vi "探头窗口-12.vi"() -> ()   [LabVIEW 2017]
panel:
  in  "更新数据":T1
  in  "停止信号":bool=TRUE
  out "更新数据？":bool=TRUE
  out "引用-切回列表模式？":refnum<vi>
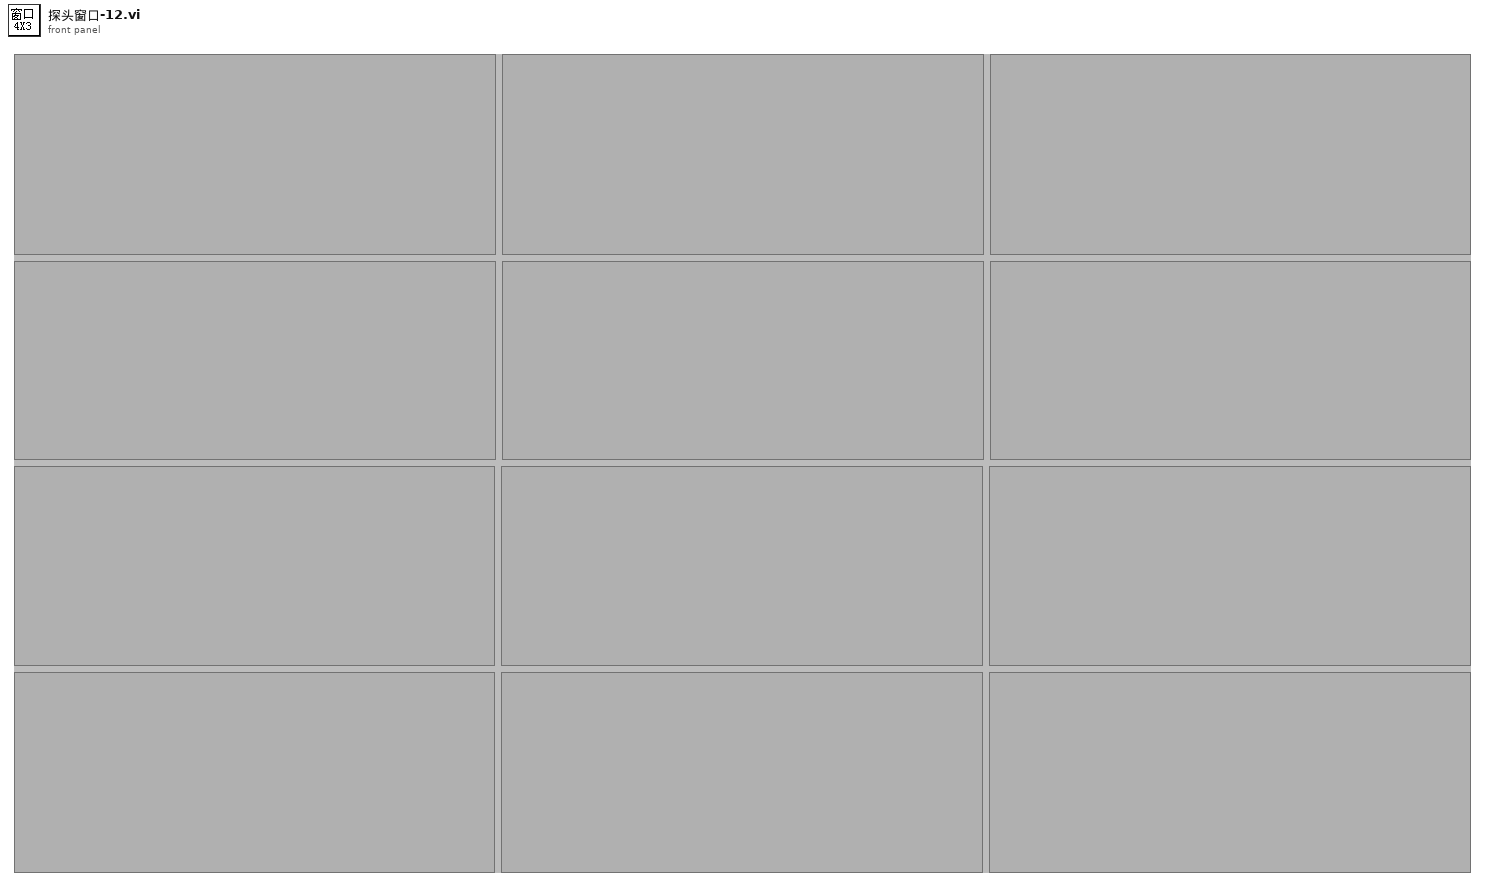
[diagram p1: front panel]
types:
  T1 = cluster{"探头启用状态？":bool[], "测量值":cluster{"X":timestamp, "Y":dbl}[], "限值":cluster{"限值1":dbl, "限值2":dbl, "探头限值":enum16{"一级限值", "二级限值"}}[], "报警状态":enum16{"正常", "一级报警", "二级报警", "累积报警"}[], "探头信息":string[], "累积剂量":cluster{"设备名称":string, "启用累积？":bool, "起始时间":timestamp, "累积剂量":dbl, "累积报警阈值":dbl}[]}
  T2 = cluster{"启用状态？":bool, "测量值":cluster{"X":timestamp, "Y":dbl}, "限值簇":cluster{"限值1":dbl, "限值2":dbl, "探头限值":enum16{"一级限值", "二级限值"}}, "报警状态":enum16{"正常", "一级报警", "二级报警", "累积报警"}, "探头信息":string, "探头地址":i32, "累积剂量":cluster{"设备名称":string, "启用累积？":bool, "起始时间":timestamp, "累积剂量":dbl, "累积报警阈值":dbl}}
  T3 = cluster{"限值1":dbl, "限值2":dbl, "探头限值":enum16{"一级限值", "二级限值"}}
  T4 = cluster{"限值1":dbl, "限值2":dbl, "探头限值":enum16{"一级限值", "二级限值"}}[]
  T5 = cluster{"设备名称":string, "启用累积？":bool, "起始时间":timestamp, "累积剂量":dbl, "累积报警阈值":dbl}[]
  T6 = cluster{"设备名称":string, "启用累积？":bool, "起始时间":timestamp, "累积剂量":dbl, "累积报警阈值":dbl}
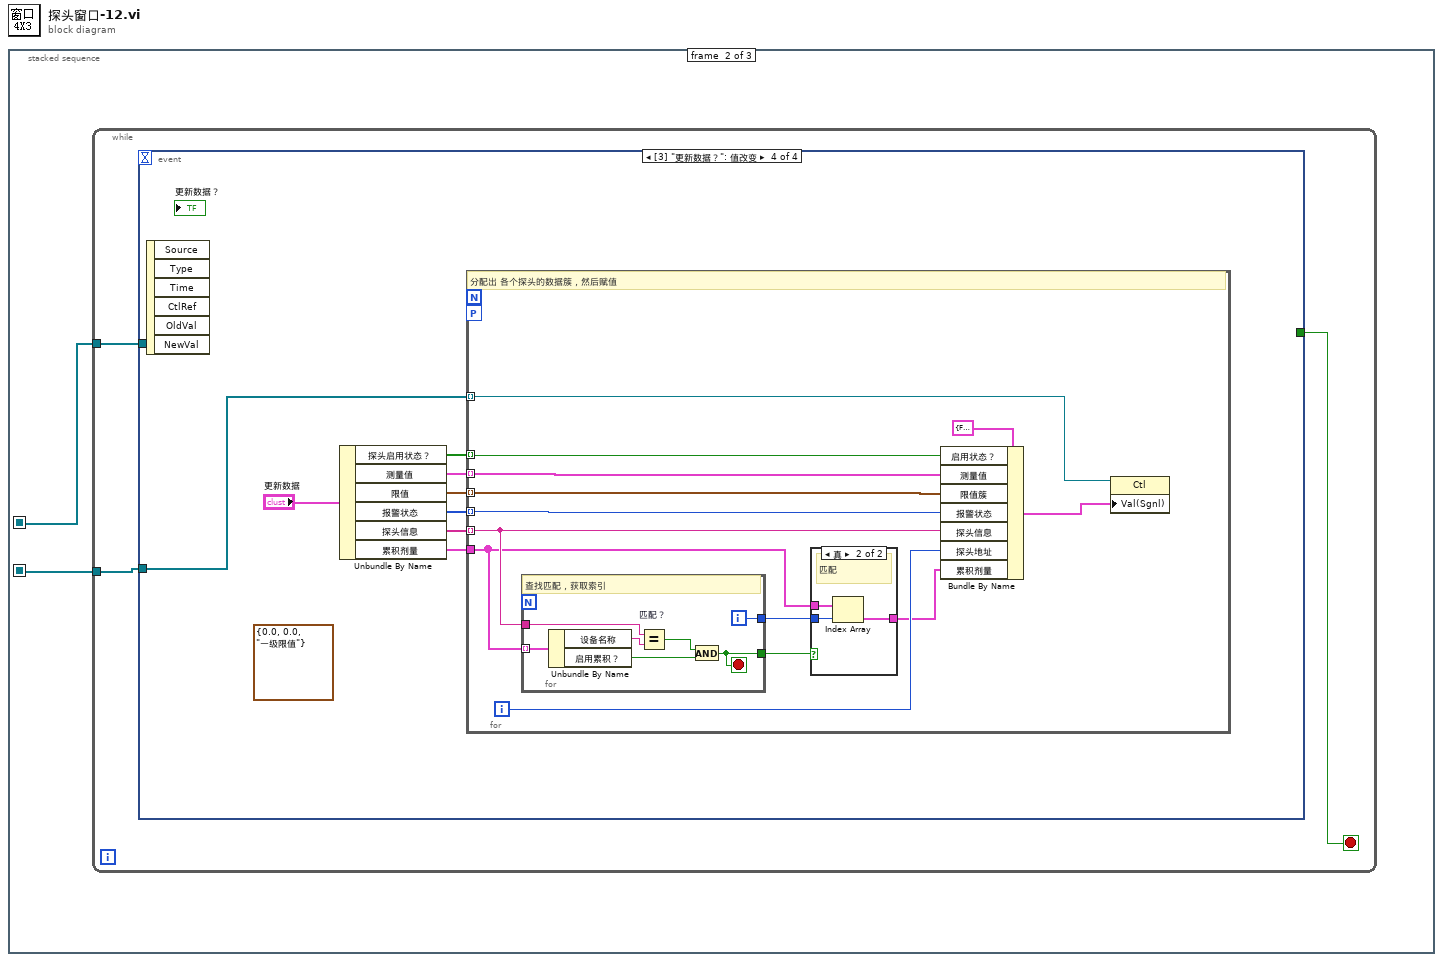
[diagram p0: block diagram]
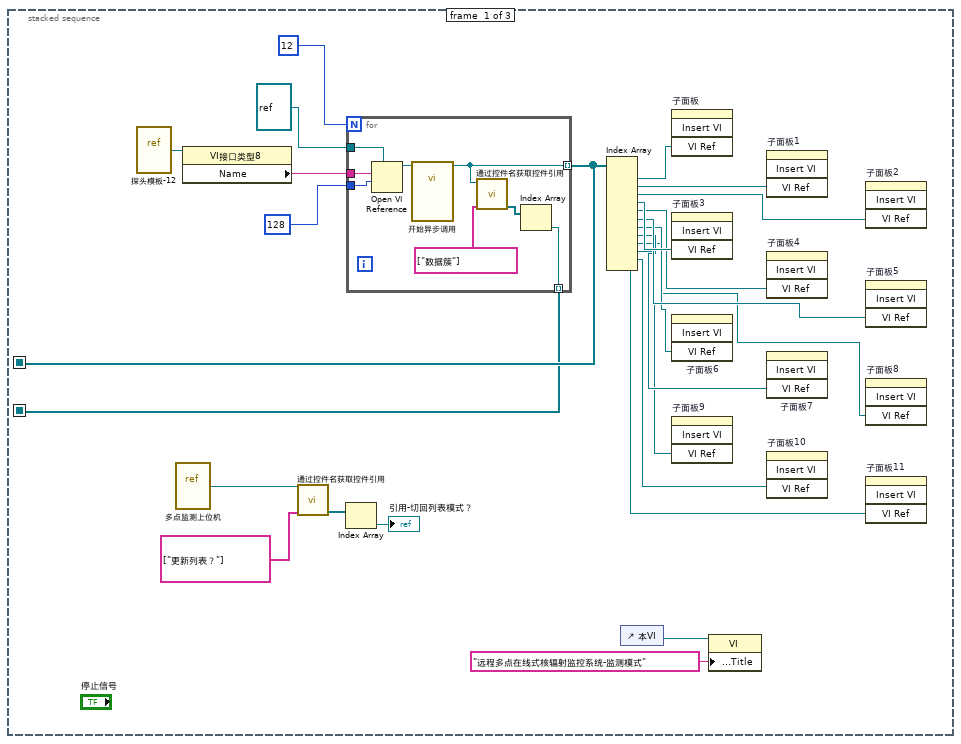
[diagram p2: hidden frame]
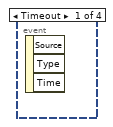
[diagram p3: hidden frame]
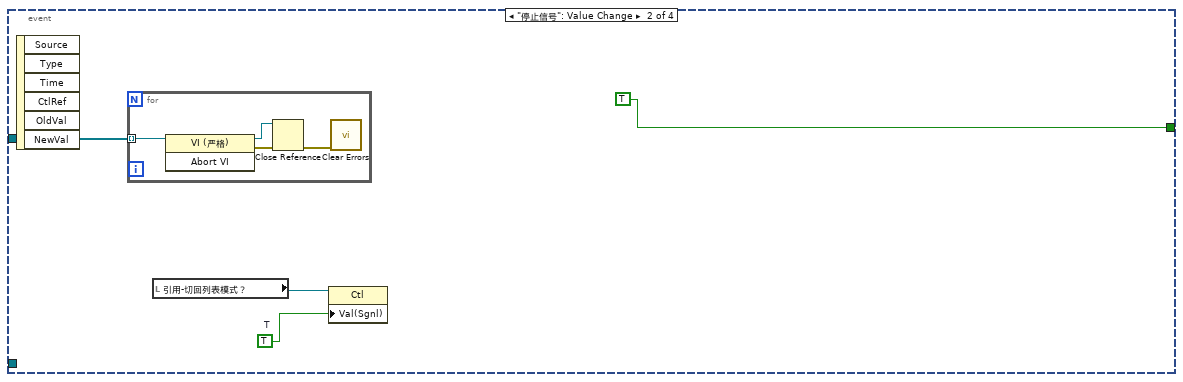
[diagram p4: hidden frame]
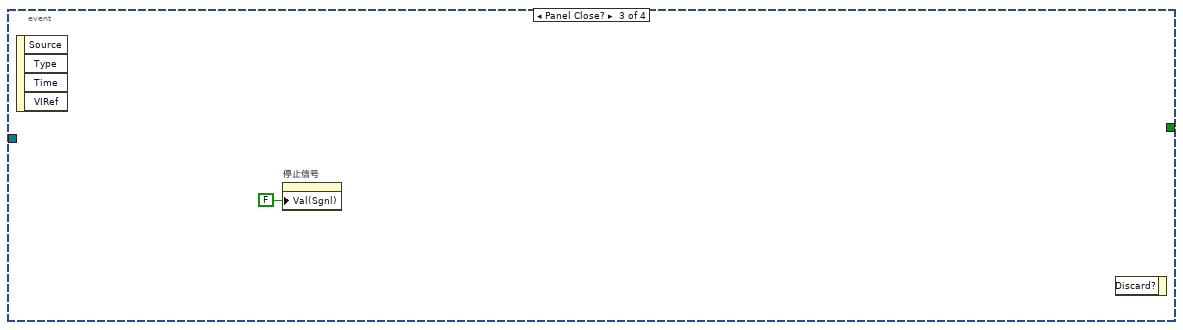
[diagram p5: hidden frame]
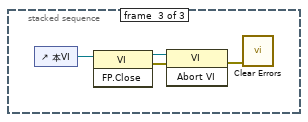
[diagram p7: hidden frame]
diagram:
  n1 = stacked-sequence {
    seq-local: [w21 _ _] -> [_ w35 _]
    seq-local: [w19 _ _] -> [_ w34 _]
    frame #0 {
      n2 = vi-ref "探头模板-12.vi"() -> (w25:refnum<vi>)
      n3 = vi-ref "多点监测上位机.vi"() -> (w3:refnum<vi>)
      n4 = property class="VI接口类型8"(reference=w25) -> ("Name"=w24:string)  [unwired: 1 in, 2 out]
      n5 = call "通过控件名获取控件引用.vi"("控件名数组"=string[] ["更新列表？"], "VI引用"=w3) -> ("控件引用输出"=w5:refnum<vi>[])  [unwired: 7 in, 2 out]
      n6 = Index Array(array=w5) -> (element=→"引用-切回列表模式？":refnum<vi>)  [unwired: 1 in]
      n7 = for {
        N: 12 -> [_]
        tunnel: w24 -> [w33]
        tunnel: 128 ("选项") -> [w32]
        tunnel: refnum<vi> refnum ("类型说明符VI引用句柄（仅用于类型）") -> [w31]
        tunnel: [w26] -> w21 mode=indexing
        tunnel: [w27] -> w19 mode=indexing
        n8 = Open VI Reference(type specifier VI Refnum (for type only)=w31, vi path=w33, options=w32) -> (vi reference=w28:refnum<vi>)  [unwired: 3 in, 1 out]
        n9 = call-by-ref "开始异步调用"(reference=w28) -> (reference out=w26:refnum<vi>)  [unwired: 13 in, 1 out]
        n10 = call "通过控件名获取控件引用.vi"("控件名数组"=string[] ["数据簇"], "VI引用"=w26) -> ("控件引用输出"=w30:refnum<vi>[])  [unwired: 7 in, 2 out]
        n11 = Index Array(array=w30) -> (element=w27:refnum<vi>)  [unwired: 1 in]
      }
      n12 = Index Array(array=w21) -> (element #1=w18:refnum<vi>, element #2=w17:refnum<vi>, element #3=w16:refnum<vi>, element #4=w15:refnum<vi>, element #5=w14:refnum<vi>, element #6=w13:refnum<vi>, element #7=w12:refnum<vi>, element #8=w11:refnum<vi>, element #9=w10:refnum<vi>, element #10=w9:refnum<vi>, element #11=w8:refnum<vi>, element #12=w7:refnum<vi>)  [unwired: 12 in]
      n13 = control-ref of="本VI"() -> (w2:refnum<vi>)
      n14 = invoke on="子面板" class="子面板" method="Insert VI"("VI Ref"=w18) -> ()  [unwired: 3 in, 4 out]
      n15 = invoke on="子面板3" class="SubPnl" method="Insert VI"("VI Ref"=w15) -> ()  [unwired: 3 in, 4 out]
      n16 = invoke on="子面板6" class="SubPnl" method="Insert VI"("VI Ref"=w12) -> ()  [unwired: 3 in, 4 out]
      n17 = invoke on="子面板9" class="SubPnl" method="Insert VI"("VI Ref"=w9) -> ()  [unwired: 3 in, 4 out]
      n18 = property class="VI"(reference=w2, "Front Panel.Title"="远程多点在线式核辐射监控系统-监测模式" ("前面板窗口:标题")) -> ()  [unwired: 1 in, 2 out]
      n19 = invoke on="子面板1" class="SubPnl" method="Insert VI"("VI Ref"=w17) -> ()  [unwired: 3 in, 4 out]
      n20 = invoke on="子面板4" class="SubPnl" method="Insert VI"("VI Ref"=w14) -> ()  [unwired: 3 in, 4 out]
      n21 = invoke on="子面板7" class="SubPnl" method="Insert VI"("VI Ref"=w11) -> ()  [unwired: 3 in, 4 out]
      n22 = invoke on="子面板10" class="SubPnl" method="Insert VI"("VI Ref"=w8) -> ()  [unwired: 3 in, 4 out]
      n23 = invoke on="子面板2" class="SubPnl" method="Insert VI"("VI Ref"=w16) -> ()  [unwired: 3 in, 4 out]
      n24 = invoke on="子面板5" class="SubPnl" method="Insert VI"("VI Ref"=w13) -> ()  [unwired: 3 in, 4 out]
      n25 = invoke on="子面板8" class="SubPnl" method="Insert VI"("VI Ref"=w10) -> ()  [unwired: 3 in, 4 out]
      n26 = invoke on="子面板11" class="SubPnl" method="Insert VI"("VI Ref"=w7) -> ()  [unwired: 3 in, 4 out]
    }
    frame #1 {
      n27 = while {
        tunnel: w35 -> [w37]
        tunnel: w34 -> [w36]
        stop <- w38 stop-if-true
        n28 = event shown="[3] \"更新数据？\": 值改变" {
          selector: _ -> [_ _ _ _]
          dyn-events: _ -> [_ _ _ _]
          timeout: _ -> [_ _ _ _]
          tunnel: [_ TRUE ("放弃？") _ _] -> w38
          tunnel: w37 -> [_ w41 _ _]
          tunnel: w36 -> [_ _ _ w48]
          event Timeout {
            n29 = event-data() -> ()  [unwired: 1 in, 3 out]
          }
          event "停止信号": Value Change {
            w39 = TRUE  # T
            n30 = event-data() -> ()  [unwired: 1 in, 6 out]
            n31 = for {
              tunnel: w41 -> [w46] mode=indexing
              n32 = invoke class="VI (严格)" method="Abort VI"(reference=w46) -> (reference out=w44:refnum<vi>, error out=w45:errorcluster)  [unwired: 2 in, 1 out]
              n33 = Close Reference(reference=w44, error in (no error)=w45) -> (error out=w43:errorcluster)
              n34 = call <vilib>:"Clear Errors.vi"("error in (no error)"=w43) -> ()  [unwired: 5 in, 2 out]
            }
            n35 = local read "引用-切回列表模式？"() -> (w40:refnum<vi>)
            n36 = property class="Ctl"(reference=w40, "Val(Sgnl)"=w39) -> ()  [unwired: 1 in, 2 out]
          }
          event Panel Close? {
            n37 = event-data() -> ()  [unwired: 1 in, 4 out]
            n38 = property on="停止信号" class="Bool (严格)"("Val(Sgnl)"=FALSE ("值(信号)")) -> ()  [unwired: 2 in, 2 out]
            n39 = event-data() -> ()  [unwired: 2 in, 1 out]
          }
          event "更新数据？": Value Change {
            (unwired) T3 {"限值1"=0.0, "限值2"=0.0, "探头限值"=enum."一级限值"} ("探头限值簇")
            n40 = event-data() -> ()  [unwired: 1 in, 6 out]
            n41 = Unbundle By Name("更新数据") -> ("探头启用状态？"=w49:bool[], "测量值"=w50:cluster{"X":timestamp, "Y":dbl}[], "限值"=w51:T4, "报警状态"=w52:enum16{"正常", "一级报警", "二级报警", "累积报警"}[], "探头信息"=w53:string[], "累积剂量"=w54:T5)
            n42 = for {
              tunnel: w49 -> [w68] mode=indexing
              tunnel: w50 -> [w67] mode=indexing
              tunnel: w51 -> [w66] mode=indexing
              tunnel: w52 -> [w65] mode=indexing
              tunnel: w53 -> [w60] mode=indexing
              workers-P: _ -> [_]
              tunnel: w48 -> [w63] mode=indexing
              tunnel: w54 -> [w59]
              i -> [w61]
              # "分配出 各个探头的数据簇，然后赋值"
              n43 = for {
                tunnel: w59 -> [w78] mode=indexing
                tunnel: w60 -> [w76]
                tunnel: [w73] -> w58
                tunnel: [w72] -> w57
                i -> [w73]
                stop <- w72 stop-if-true
                # "查找匹配，获取索引"
                n44 = Unbundle By Name(w78) -> ("设备名称"=w77:string, "启用累积？"=w74:bool)
                n45 = Equal? "匹配？"(x=w76, y=w77) -> (x = y?=w75:bool)
                n46 = And(x=w75, y=w74) -> (x .and. y?=w72:bool)
              }
              n47 = case shown="真" w57 {
                tunnel: w59 -> [_ w71]
                tunnel: w58 -> [_ w70]
                tunnel: [_ w69] -> w56
                frame False {
                  # "不匹配"
                }
                frame True {
                  # "匹配"
                  n48 = Index Array(array=w71, index=w70) -> (element=w69:T6)
                }
              }
              n49 = Bundle By Name(cluster=T2 {"启用状态？"=FALSE, "测量值"={"X"=timestamp(0 s since 1904-01-01), "Y"=0.0}, "限值簇"={"限值1"=0.0, "限值2"=0.0, "探头限值"=enum."一级限值"}, "报警状态"=enum."正常", "探头信息"="", "探头地址"=0, "累积剂量"={"设备名称"="", "启用累积？"=FALSE, "起始时间"=timestamp(0 s since 1904-01-01), "累积剂量"=0.0, "累积报警阈值"=0.0}} ("输出簇"), "启用状态？"=w68, "测量值"=w67, "限值簇"=w66, "报警状态"=w65, "探头信息"=w60, "探头地址"=w61, "累积剂量"=w56) -> (w62:T2)
              n50 = property class="Ctl"(reference=w63, "Val(Sgnl)"=w62) -> ()  [unwired: 1 in, 2 out]
            }
          }
        }
      }
    }
    frame #2 {
      n51 = control-ref of="本VI"() -> (w82:refnum<vi>)
      n52 = invoke class="VI" method="FP.Close"(reference=w82) -> (reference out=w81:refnum<vi>, error out=w80:errorcluster)  [unwired: 2 in, 1 out]
      n53 = invoke class="VI" method="Abort VI"(reference=w81, error in=w80) -> (error out=w79:errorcluster)  [unwired: 1 in, 2 out]
      n54 = call <vilib>:"Clear Errors.vi"("error in (no error)"=w79) -> ()  [unwired: 5 in, 2 out]
    }
  }
